vi "客户端侦听列表.vi"() -> ()   [LabVIEW 2016, in "wxpusher.lvlib"]
uses:
  wxpusher.lvlib
  <vilib>/Utility/miscctls.llb/LVPointTypeDef.ctl
  <vilib>/httpClient/LabVIEWHTTPClient.lvlib
panel:
  out "有效回调":refnum<k5>[](array[refnum])
  out "有效主机列表":T1(array[cluster])
  out "长度":i32
  out "错误输出":errorcluster
  out "数据输出":string
  in  "开机启动":bool
  out "remote port":u16
  out "remote address":string
  out "data out":string
  out "新增回调":refnum<k5>[](array[refnum])
  out "回调信息":T2
  out "新增主机列表":T1(array[cluster])
  in  "客户端列表":i32(listbox)
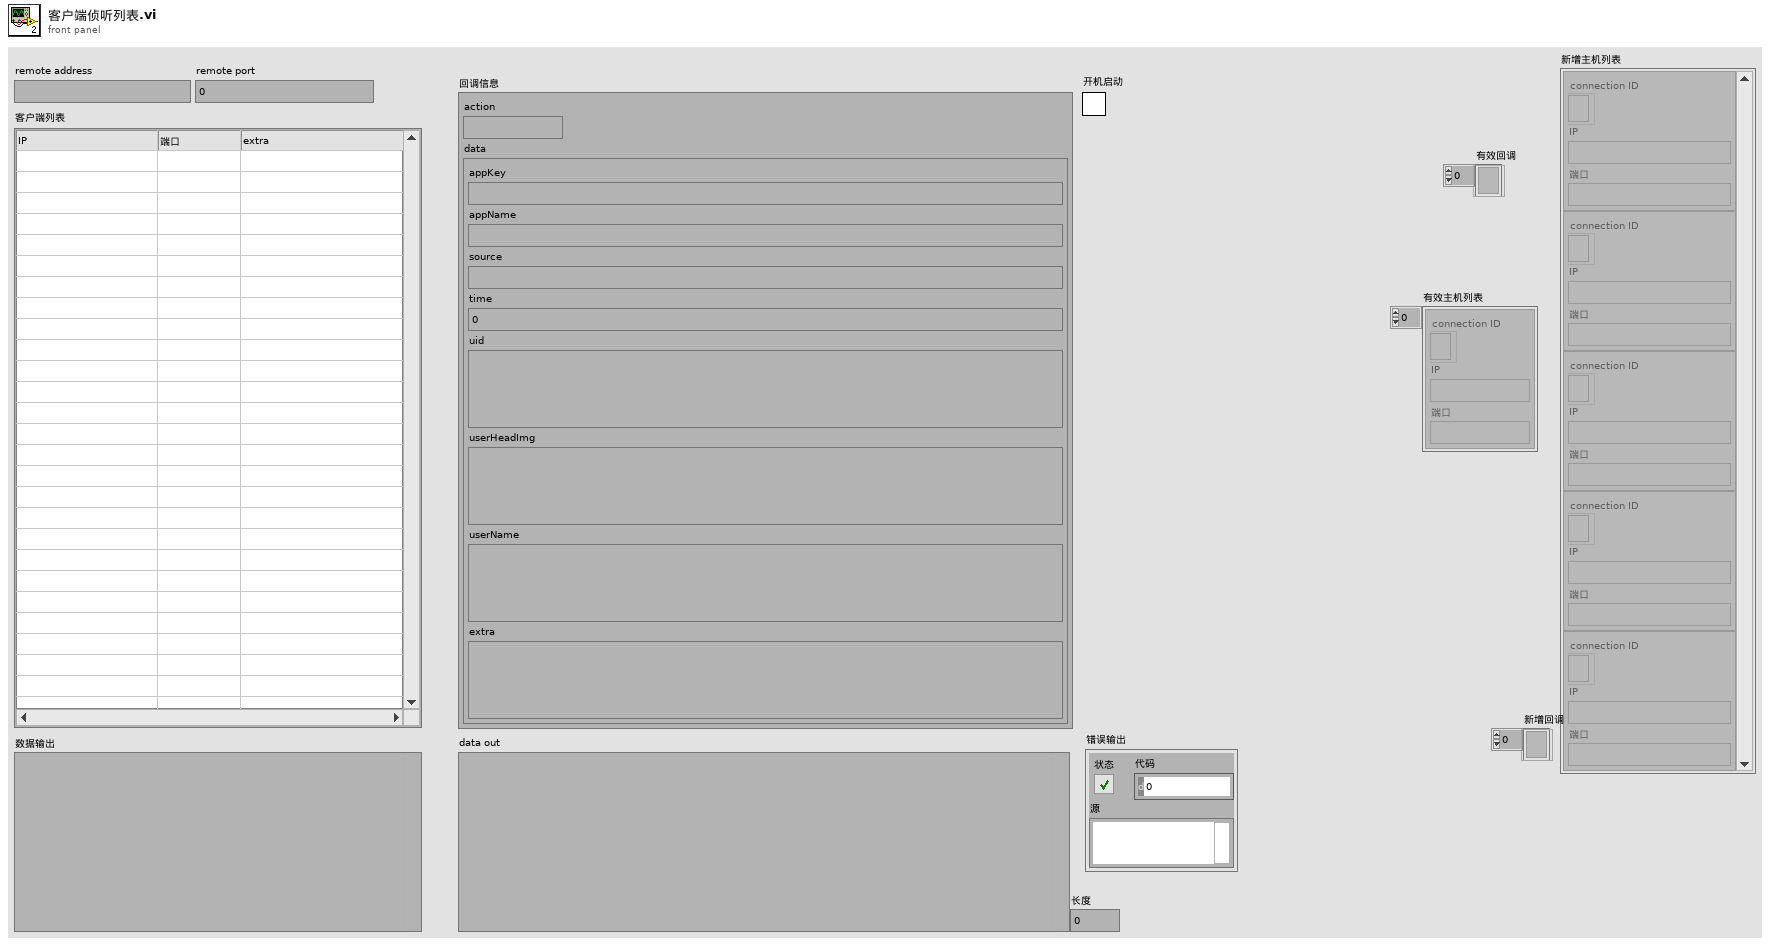
[diagram p1: front panel]
types:
  T1 = cluster{"connection ID":refnum<k5>, "IP":string, "端口":string}[]
  T2 = cluster{"action":string, "data":cluster{"appKey":string, "appName":string, "source":string, "time":u64, "uid":string, "userHeadImg":string, "userName":string, "extra":string}}
  T3 = typedef "LVPointTypeDef.ctl" = cluster{"Horizontal":i16, "Vertical":i16}
  T4 = cluster{"数据输出":string, "data":cluster{"action":string, "data":cluster{"appKey":string, "appName":string, "source":string, "time":u64, "uid":string, "userHeadImg":string, "userName":string, "extra":string}}}
  T5 = cluster{"connection ID":refnum<k5>, "IP":string, "端口":string}
  T6 = enum16{"Standard", "Buffered", "CRLF", "Immediate"}
  T7 = cluster{"cmd":string, "data":cluster{"png":u8[]}}
  T8 = typedef "LabVIEWHTTPClient.lvlib/ClientHandle.ctl" = refnum<k1>
  T9 = cluster{"data out":string, "类型和默认值":cluster{"action":string, "data":cluster{"appKey":string, "appName":string, "source":string, "time":u64, "uid":string, "userHeadImg":string, "userName":string, "extra":string}}}
  T10 = cluster{"cmd":string, "data":cluster{"action":string, "data":cluster{"appKey":string, "appName":string, "source":string, "time":u64, "uid":string, "userHeadImg":string, "userName":string, "extra":string}}}
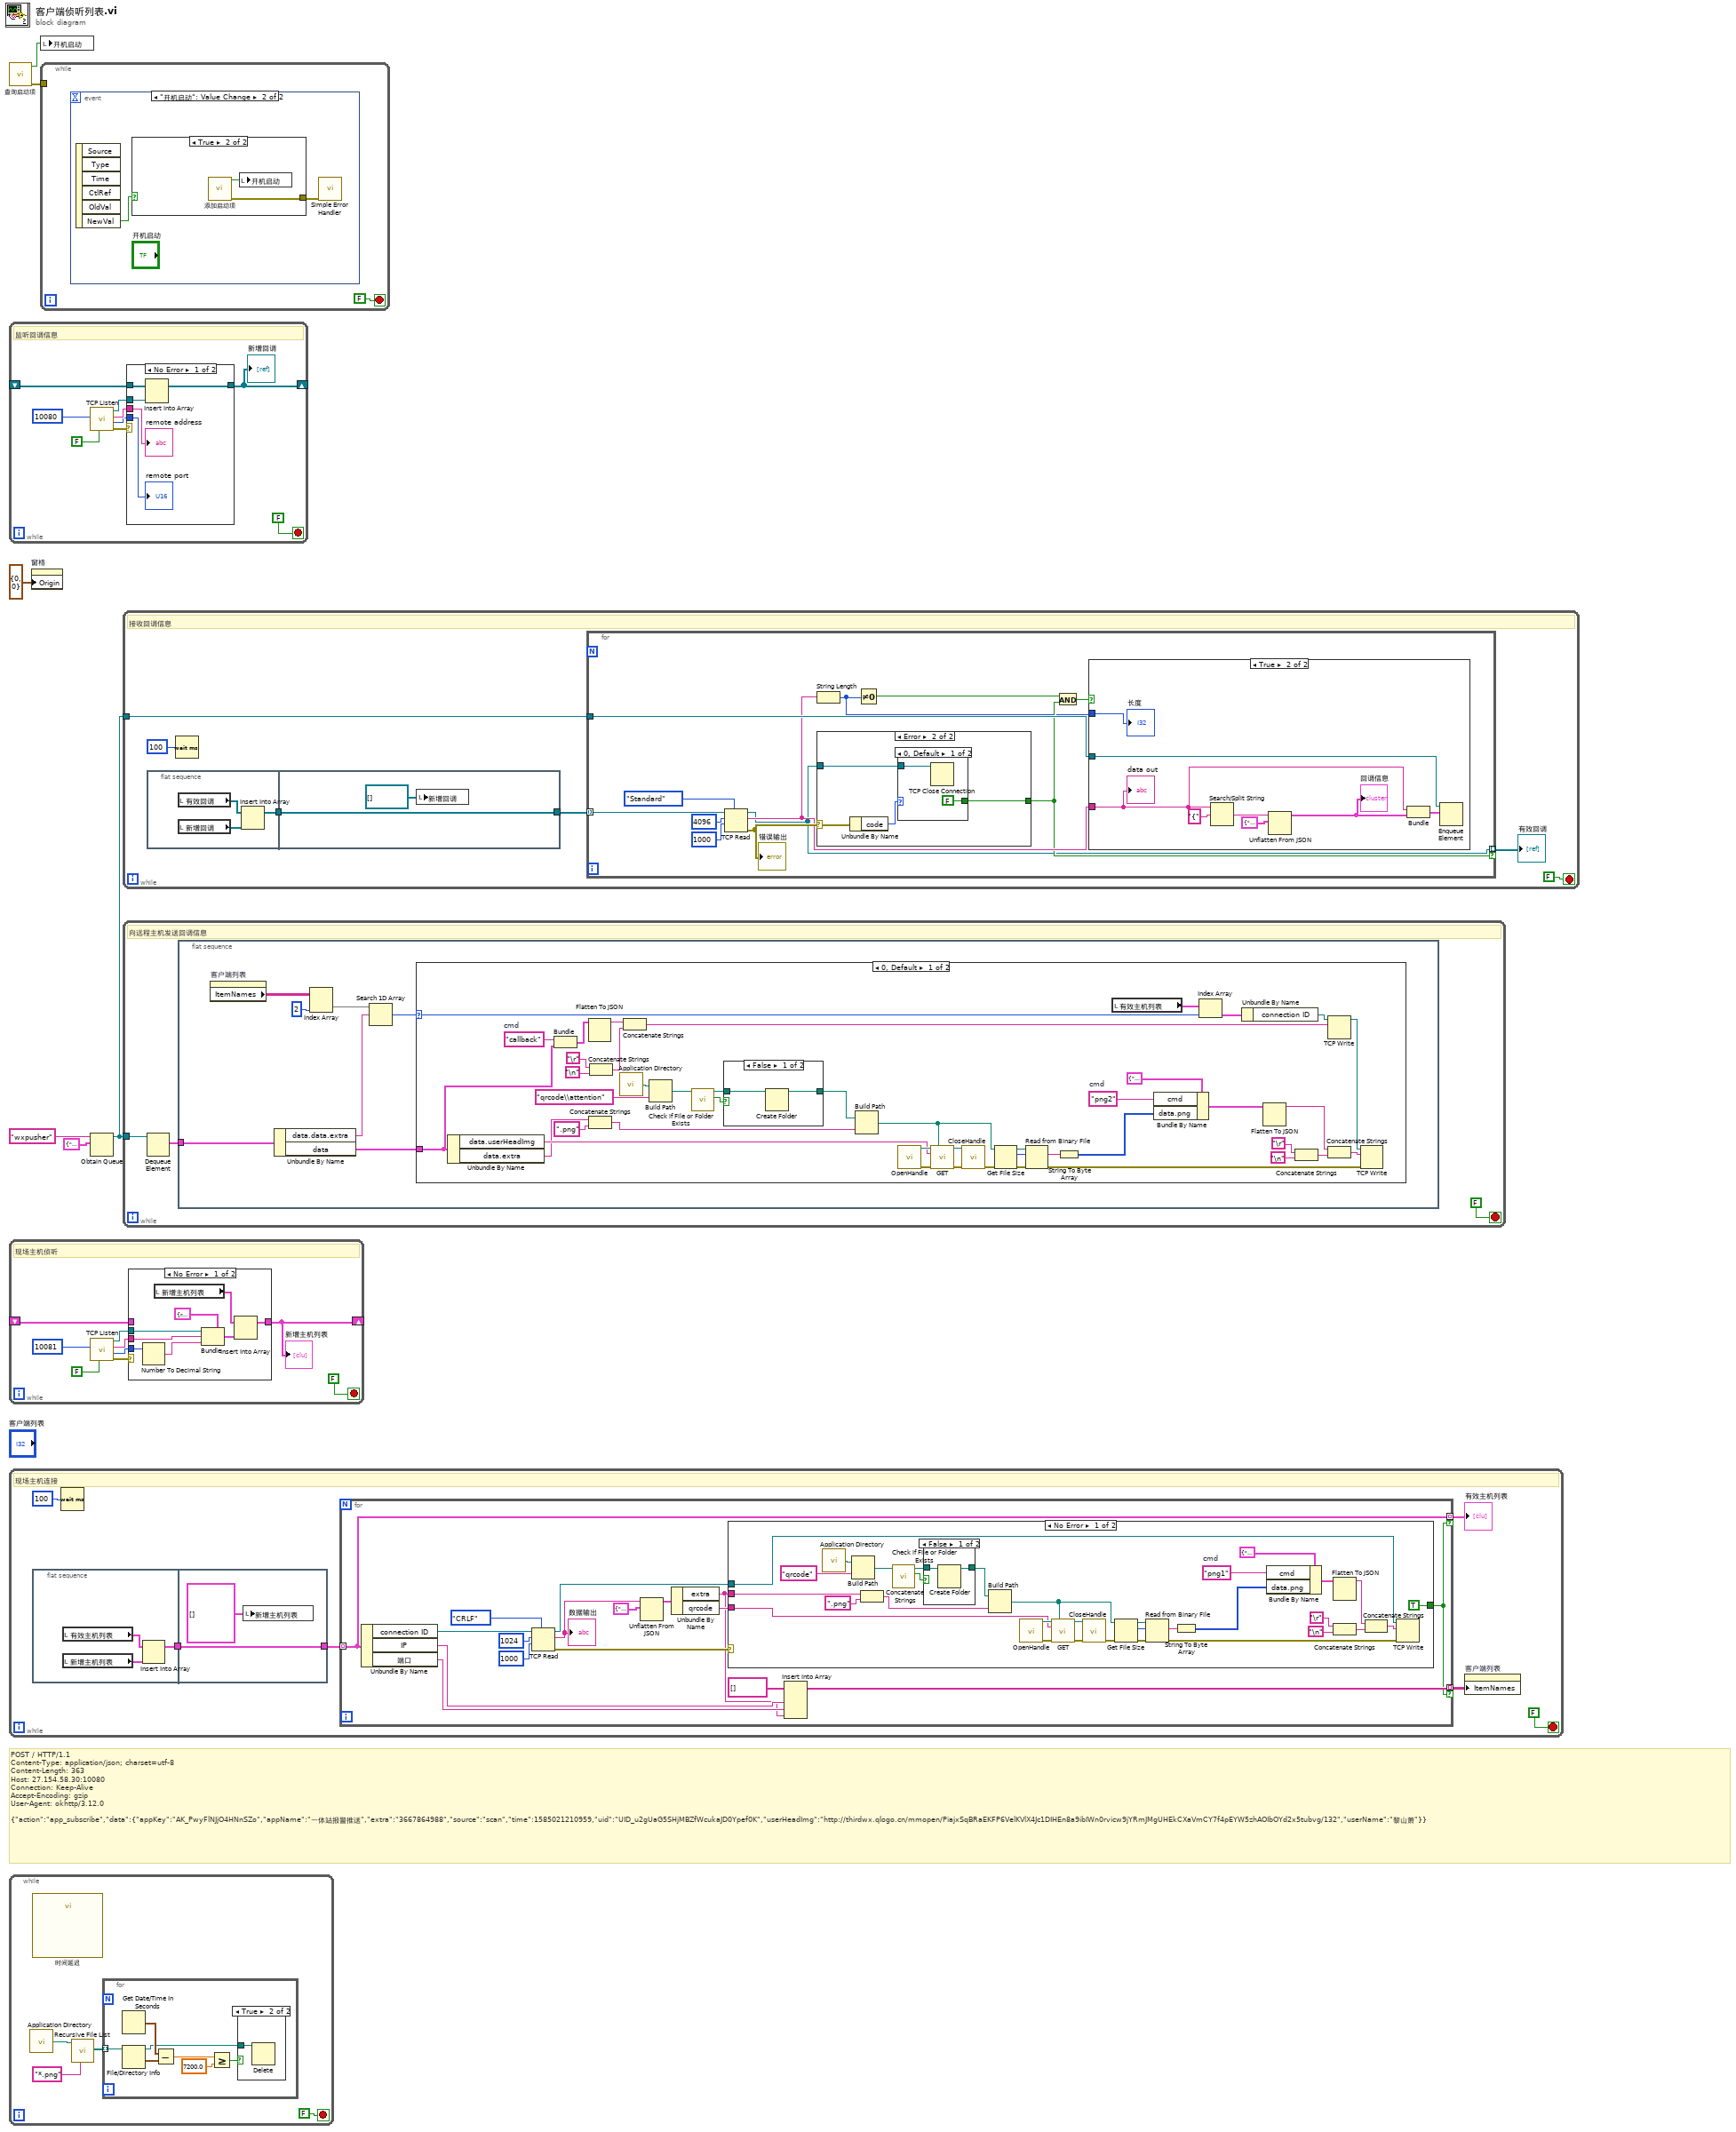
[diagram p0: block diagram]
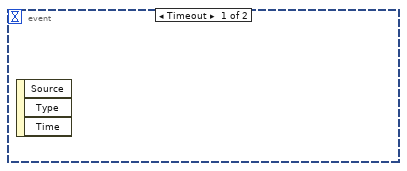
[diagram p3: hidden frame]
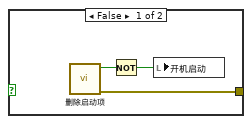
[diagram p4: hidden frame]
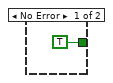
[diagram p6: hidden frame]
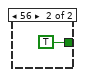
[diagram p7: hidden frame]
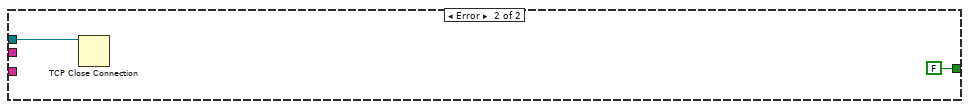
[diagram p12: hidden frame]
diagram:
  # "POST / HTTP/1.1\nContent-Type: application/json; charset=utf-8\nContent-Length: 363\nHost: 27.154.58.30:10080\nConnection: Keep-Alive\nAccept-Encoding: gzip\nUser-Agent: okhttp/3.12.0\n\n{\"action\":\"app_subscribe\",\"data\":{\"appKey\":\"AK_PwyFlNJjO4HNnSZo\",\"appName\":\"一体站报警推送\",\"extra\":\"3667864988\",\"source\":\"scan\",\"time\":1585021210959,\"uid\":\"UID_u2gUaG5SHjMBZfWcukaJD0Ypef0K\",\"userHeadImg\":\"http://thirdwx.qlogo.cn/mmopen/PiajxSqBRaEKFP6VelKVlX4Jc1DIHEn8a9ibIWn0rvicw9jYRmJMgUHEkCXaVmCY7f4pEYW5zhAOIbOYd2x5tubvg/132\",\"userName\":\"黎山萧\"}}"
  n1 = call "查询启动项.vi"() -> ("error out"=w3:errorcluster, "包含启动项"=w2:bool)  [unwired: 9 in, 1 out]
  n2 = while {
    shift-right: [w10] -> _
    shift-left: _ -> [w9]
    stop <- FALSE stop-if-true
    # "监听回调信息"
    n3 = call <vilib>:"TCP Listen.vi"("resolve remote address (T)"=FALSE, "port"=u16 10080) -> ("error out"=w13:errorcluster, "remote port"=w7:u16, "remote address"=w12:string, "connection ID"=w11:refnum<k5>)  [unwired: 5 in, 1 out]
    n4 = case shown="No Error" w13 {
      tunnel: w11 -> [w20 _]
      tunnel: w12 -> [w17 _]
      tunnel: [w19 w21] -> w10
      tunnel: w9 -> [w18 w21]
      tunnel: w7 -> [w16 _]
      frame No Error {
        n5 = Insert Into Array(array=w18, new element=w20) -> (w19:refnum<k5>[])  [unwired: 1 in]
        "remote address" <- w17
        "remote port" <- w16
      }
      frame Error {
      }
    }
    "新增回调" <- w10
  }
  n6 = while {
    shift-right: [w24] -> _
    shift-left: _ -> [w23]
    stop <- FALSE stop-if-true
    # "现场主机侦听"
    n7 = call <vilib>:"TCP Listen.vi"("resolve remote address (T)"=FALSE, "port"=u16 10081) -> ("error out"=w28:errorcluster, "remote port"=w25:u16, "remote address"=w26:string, "connection ID"=w27:refnum<k5>)  [unwired: 5 in, 1 out]
    n8 = case shown="No Error" w28 {
      tunnel: w27 -> [w38 _]
      tunnel: w26 -> [w32 _]
      tunnel: w25 -> [w33 _]
      tunnel: [w36 w39] -> w24
      tunnel: w23 -> [_ w39]
      frame No Error {
        n9 = Number To Decimal String(number=w33) -> (decimal integer string=w35:string)  [unwired: 1 in]
        n10 = local read "新增主机列表"() -> (w31:T1)
        n11 = Bundle(cluster=T5 {"connection ID"=refnum, "IP"="", "端口"=""} ("簇"), "connection ID"=w38, "IP"=w32, "端口"=w35) -> (w37:T5)
        n12 = Insert Into Array(array=w31, new element=w37) -> (w36:T1)  [unwired: 1 in]
      }
      frame Error {
      }
    }
    "新增主机列表" <- w24
  }
  n13 = while {
    stop <- FALSE stop-if-true
    # "现场主机连接"
    n14 = flat-sequence {
      tunnel: [w46] -> w40
      tunnel: [w50] -> w42
      tunnel: w40 -> [w50]
      frame #0 {
        n15 = local read "有效主机列表"() -> (w47:T1)
        n16 = local read "新增主机列表"() -> (w48:T1)
        n17 = Insert Into Array(array=w47, new element=w48) -> (w46:T1)  [unwired: 1 in]
      }
      frame #1 {
        n18 = local write "新增主机列表"(T1 [] ("新增主机列表")) -> ()
      }
    }
    n19 = Wait (ms)(milliseconds to wait=u32 100 ("等待时间（毫秒）")) -> ()  [unwired: 1 out]
    n20 = for {
      tunnel: w42 -> [w56] mode=indexing
      tunnel: [w61] -> w43 mode=indexing if=w55
      tunnel: [w56] -> w41 mode=indexing if=w55
      n21 = Unbundle By Name(w56) -> ("connection ID"=w67:refnum<k5>, "IP"=w64:string, "端口"=w63:string)
      n22 = TCP Read(connection ID=w67, bytes to read=1024 ("读取的字节"), 7:T6."CRLF" ("模式（标准）"), 9:1000 ("超时毫秒(25000)")) -> (connection ID out=w54:refnum<k5>, data out=w59:string, error out=w60:errorcluster)  [unwired: 1 in]
      "数据输出" <- w59
      n23 = Unflatten From JSON(JSON string=w59, type and defaults=cluster{"extra":string, "qrcode":string} {"extra"="", "qrcode"=""}) -> (value=w57:cluster{"extra":string, "qrcode":string})  [unwired: 5 in, 1 out]
      n24 = Unbundle By Name(w57) -> ("extra"=w52:string, "qrcode"=w53:string)
      n25 = case shown="No Error" w60 {
        tunnel: [TRUE FALSE] -> w55
        tunnel: w54 -> [w70 w103]
        tunnel: w53 -> [w69 _]
        tunnel: w52 -> [w68 _]
        frame No Error {
          w96 = "png1"  # cmd
          n26 = call <vilib>:"Application Directory.vi"() -> ("Application Directory"=w88:path)
          n27 = Build Path(base path=w88, name or relative path="qrcode" ("名称或相对路径")) -> (appended path=w76:path)
          n28 = Concatenate Strings(w68, ".png" ("字符串")) -> (w81:string)
          n29 = call <vilib>:"Check if File or Folder Exists.vi"("path"=w76) -> ("file or folder exists?"=w78:bool, "dup path"=w77:path)  [unwired: 8 in, 1 out]
          n30 = case shown="False" w78 {
            tunnel: [w101 w102] -> w75
            tunnel: w77 -> [w100 w102]
            frame False {
              n31 = Create Folder(path (use dialog)=w100) -> (created path=w101:path)  [unwired: 2 in, 2 out]
            }
            frame True {
            }
          }
          n32 = Build Path(base path=w75, name or relative path=w81) -> (appended path=w82:path)
          n33 = call <vilib>:"OpenHandle.vi"() -> ("client handle out"=w71:T8, "error out"=w72:errorcluster)  [unwired: 14 in]
          n34 = call <vilib>:"GET.vi"("client handle"=w71, "output file"=w82, "url"=w69, "error in (no error)"=w72) -> ("client handle out"=w73:T8, "error out"=w74:errorcluster)  [unwired: 8 in, 2 out]
          n35 = call <vilib>:"CloseHandle.vi"("client handle"=w73, "error in (no error)"=w74) -> ("error out"=w84:errorcluster)  [unwired: 13 in]
          n36 = Get File Size(file=w82, error in=w84) -> (refnum out=w83:refnum<file>, size (in bytes)=w86:i64, 0:w85:errorcluster)
          n37 = Read from Binary File(8:w85, 10:w86, 11:w83) -> (0:w87:errorcluster, 2:w97:string)  [unwired: 3 in, 2 out]
          n38 = String To Byte Array(string=w97) -> (unsigned byte array=w98:u8[])
          n39 = Bundle By Name(cluster=T7 {"cmd"="", "data"={"png"=[]}}, "cmd"=w96, "data.png"=w98) -> (w90:T7)
          n40 = Flatten To JSON(anything=w90) -> (JSON string=w91:string)  [unwired: 2 in, 1 out]
          n41 = Concatenate Strings("\r", "\n") -> (w95:string)
          n42 = Concatenate Strings(w91, w95) -> (w92:string)
          n43 = TCP Write(connection ID=w70, data in=w92, error in (no error)=w87) -> ()  [unwired: 1 in, 3 out]
        }
        frame Error {
          n44 = TCP Close Connection(connection ID=w103) -> ()  [unwired: 2 in, 2 out]
        }
      }
      n45 = Insert Into Array(array=string[] [] ("数组"), new element #1=w64, new element #2=w63, new element #3=w52) -> (w61:string[])  [unwired: 1 in]
    }
    "有效主机列表" <- w41
    n46 = property on="客户端列表" class="MCListbox (strict)"("ItemNames"=w43) -> ()  [unwired: 2 in, 2 out]
  }
  n47 = while {
    stop <- FALSE stop-if-true
    n48 = call <vilib>:"Application Directory.vi"() -> ("Application Directory"=w107:path)
    n49 = call "时间延迟"() -> ()  [unwired: 11 in, 1 out]
    n50 = call <vilib>:"Recursive File List.vi"("pattern"="*.png", "Folder Path"=w107) -> ("All Files in Dir"=w105:path[])  [unwired: 5 in, 4 out]
    n51 = for {
      tunnel: w105 -> [w115] mode=indexing
      n52 = Get Date/Time In Seconds() -> (seconds since 1Jan1904=w113:timestamp)
      n53 = File/Directory Info(path=w115) -> (path out=w109:path, last mod=w114:timestamp)  [unwired: 1 in, 5 out]
      n54 = Subtract(x=w113, y=w114) -> (x-y=w112:dbl)
      n55 = Greater Or Equal?(x=w112, y=7200.0) -> (x >= y?=w110:bool)
      n56 = case shown="True" w110 {
        tunnel: w109 -> [_ w116]
        frame False {
        }
        frame True {
          n57 = Delete(path (use dialog)=w116) -> ()  [unwired: 4 in, 3 out]
        }
      }
    }
  }
  n58 = property on="窗格" class="Pane"("Origin"=T3 {"Horizontal"=0, "Vertical"=0} ("原点")) -> ()  [unwired: 2 in, 2 out]
  n59 = local write "开机启动"(w2) -> ()
  n60 = while {
    tunnel: w3 -> [_]
    stop <- FALSE stop-if-true
    n61 = event shown="[1] \"开机启动\": Value Change" {
      selector: _ -> [_ _]
      dyn-events: _ -> [_ _]
      timeout: _ -> [_ _]
      event Timeout {
        n62 = event-data() -> ()  [unwired: 1 in, 3 out]
      }
      event "开机启动": Value Change {
        n63 = event-data() -> ("NewVal"=w119:bool)  [unwired: 1 in, 5 out]
        n64 = case shown="True" w119 {
          tunnel: [w120 w123] -> w118
          frame False {
            n65 = call "删除启动项.vi"() -> ("error out"=w120:errorcluster, "删除标记"=w122:bool)  [unwired: 10 in]
            n66 = Not(x=w122) -> (.not. x?=w121:bool)
            n67 = local write "开机启动"(w121) -> ()
          }
          frame True {
            n68 = call "添加启动项.vi"() -> ("error out"=w123:errorcluster, "添加成功标记"=w124:bool)  [unwired: 10 in]
            n69 = local write "开机启动"(w124) -> ()
          }
        }
        n70 = call <vilib>:"Simple Error Handler.vi"("error in (no error)"=w118) -> ()  [unwired: 4 in, 5 out]
      }
    }
  }
  n71 = Obtain Queue(name (unnamed)="wxpusher" ("名称（未命名）"), element data type=T4 {"数据输出"="", "data"={"action"="", "data"={"appKey"="", "appName"="", "source"="", "time"=0, "uid"="", "userHeadImg"="", "userName"="", "extra"=""}}}) -> (queue out=w4:refnum<queue>)  [unwired: 3 in, 2 out]
  n72 = while "While循环" {
    tunnel: w4 -> [w129]
    stop <- FALSE stop-if-true
    # "接收回调信息"
    n73 = flat-sequence {
      tunnel: [w131] -> w125
      tunnel: [w135] -> w126
      tunnel: w125 -> [w135]
      frame #0 {
        n74 = local read "有效回调"() -> (w133:refnum<k5>[])
        n75 = local read "新增回调"() -> (w132:refnum<k5>[])
        n76 = Insert Into Array(array=w133, new element=w132) -> (w131:refnum<k5>[])  [unwired: 1 in]
      }
      frame #1 {
        n77 = local write "新增回调"(refnum<k5>[] [] ("新增回调")) -> ()
      }
    }
    n78 = Wait (ms)(milliseconds to wait=u32 100 ("等待时间（毫秒）")) -> ()  [unwired: 1 out]
    n79 = for {
      tunnel: w129 -> [w147]
      tunnel: w126 -> [w143] mode=indexing
      tunnel: [w137] -> w127 mode=indexing if=w138
      n80 = TCP Read(connection ID=w143, bytes to read=4096 ("读取的字节"), 7:T6."Standard" ("模式（标准）"), 9:1000 ("超时毫秒(25000)")) -> (connection ID out=w137:refnum<k5>, data out=w141:string, error out=w142:errorcluster)  [unwired: 1 in]
      "错误输出" <- w142
      n81 = String Length(string=w141) -> (length=w136:i32)
      n82 = case shown="Error" w142 {
        selector: w142 -> [_ w160]
        tunnel: [TRUE w158] -> w138
        tunnel: w137 -> [_ w157]
        frame No Error {
        }
        frame Error {
          n83 = Unbundle By Name(w160) -> ("code"=w159:i32)
          n84 = case shown="0, Default" w159 {
            tunnel: [FALSE TRUE] -> w158
            tunnel: w157 -> [w161 _]
            frame 0, Default {
              n85 = TCP Close Connection(connection ID=w161) -> ()  [unwired: 2 in, 2 out]
            }
            frame 56 {
            }
          }
        }
      }
      n86 = Not Equal To 0?(x=w136) -> (x != 0?=w139:bool)
      n87 = And(x=w139, y=w138) -> (x .and. y?=w140:bool)
      n88 = case shown="True" w140 {
        tunnel: w147 -> [_ w155]
        tunnel: w141 -> [_ w154]
        tunnel: w136 -> [_ w148]
        frame False {
        }
        frame True {
          n89 = Search/Split String(string=w154, search string/char (-)="{" ("搜索字符串/字符(-)")) -> (match + rest of string=w151:string)  [unwired: 1 in, 2 out]
          n90 = Unflatten From JSON(JSON string=w151, type and defaults=T2 {"action"="", "data"={"appKey"="", "appName"="", "source"="", "time"=0, "uid"="", "userHeadImg"="", "userName"="", "extra"=""}} ("类型和默认值")) -> (value=w150:T2)  [unwired: 5 in, 1 out]
          "回调信息" <- w150
          n91 = Bundle("data out"=w154, "类型和默认值"=w150) -> (w149:T9)  [unwired: 1 in]
          n92 = Enqueue Element(queue=w155, element=w149) -> ()  [unwired: 2 in, 3 out]
          "data out" <- w154
          "长度" <- w148
        }
      }
    }
    "有效回调" <- w127
  }
  n93 = while {
    tunnel: w4 -> [w166]
    stop <- FALSE stop-if-true
    # "向远程主机发送回调信息"
    n94 = Dequeue Element(queue=w166) -> (element=w164:T4)  [unwired: 2 in, 3 out]
    n95 = flat-sequence {
      tunnel: w164 -> [w173]
      frame #0 {
        n96 = property on="客户端列表" class="MCListbox (strict)"() -> ("ItemNames"=w172:string[][])  [unwired: 2 in, 2 out]
        n97 = Unbundle By Name(w173) -> ("data.data.extra"=w169:string, "data"=w167:T2)
        n98 = Index Array(array=w172, index (col)=2 ("禁用的索引 (列)")) -> (element=w170:string[])  [unwired: 1 in]
        n99 = Search 1D Array(1D array=w170, element=w169) -> (index of element=w168:i32)  [unwired: 1 in]
        n100 = case shown="0, Default" w168 {
          selector: w168 -> [w215 _]
          tunnel: w167 -> [w207 _]
          frame 0, Default {
            w179 = "png2"  # cmd
            w206 = "callback"  # cmd
            n101 = Unbundle By Name(w207) -> ("data.userHeadImg"=w176:string, "data.extra"=w175:string)
            n102 = Bundle("cmd"=w206, "data"=w207) -> (w205:T10)  [unwired: 1 in]
            n103 = Flatten To JSON(anything=w205) -> (JSON string=w212:string)  [unwired: 2 in, 1 out]
            n104 = Concatenate Strings(w175, ".png" ("字符串")) -> (w194:string)
            n105 = Concatenate Strings("\r", "\n") -> (w208:string)
            n106 = call <vilib>:"Application Directory.vi"() -> ("Application Directory"=w187:path)
            n107 = Concatenate Strings(w212, w208) -> (w211:string)
            n108 = Build Path(base path=w187, name or relative path="qrcode\\attention" ("名称或相对路径")) -> (appended path=w199:path)
            n109 = call <vilib>:"Check if File or Folder Exists.vi"("path"=w199) -> ("file or folder exists?"=w197:bool, "dup path"=w198:path)  [unwired: 8 in, 1 out]
            n110 = case shown="False" w197 {
              tunnel: [w218 w219] -> w200
              tunnel: w198 -> [w217 w219]
              frame False {
                n111 = Create Folder(path (use dialog)=w217) -> (created path=w218:path)  [unwired: 2 in, 2 out]
              }
              frame True {
              }
            }
            n112 = Build Path(base path=w200, name or relative path=w194) -> (appended path=w193:path)
            n113 = call <vilib>:"OpenHandle.vi"() -> ("client handle out"=w204:T8, "error out"=w203:errorcluster)  [unwired: 14 in]
            n114 = call <vilib>:"GET.vi"("client handle"=w204, "output file"=w193, "url"=w176, "error in (no error)"=w203) -> ("client handle out"=w202:T8, "error out"=w201:errorcluster)  [unwired: 8 in, 2 out]
            n115 = call <vilib>:"CloseHandle.vi"("client handle"=w202, "error in (no error)"=w201) -> ("error out"=w191:errorcluster)  [unwired: 13 in]
            n116 = Get File Size(file=w193, error in=w191) -> (refnum out=w192:refnum<file>, size (in bytes)=w189:i64, 0:w190:errorcluster)
            n117 = Read from Binary File(8:w190, 10:w189, 11:w192) -> (0:w188:errorcluster, 2:w178:string)  [unwired: 3 in, 2 out]
            n118 = String To Byte Array(string=w178) -> (unsigned byte array=w177:u8[])
            n119 = local read "有效主机列表"() -> (w216:T1)
            n120 = Bundle By Name(cluster=T7 {"cmd"="", "data"={"png"=[]}}, "cmd"=w179, "data.png"=w177) -> (w185:T7)
            n121 = Index Array(array=w216, index=w215) -> (element=w214:T5)
            n122 = Unbundle By Name(w214) -> ("connection ID"=w213:refnum<k5>)
            n123 = Flatten To JSON(anything=w185) -> (JSON string=w184:string)  [unwired: 2 in, 1 out]
            n124 = Concatenate Strings("\r", "\n") -> (w180:string)
            n125 = TCP Write(connection ID=w213, data in=w211) -> (connection ID out=w174:refnum<k5>)  [unwired: 2 in, 2 out]
            n126 = Concatenate Strings(w184, w180) -> (w183:string)
            n127 = TCP Write(connection ID=w174, data in=w183, error in (no error)=w188) -> ()  [unwired: 1 in, 3 out]
          }
          frame -1 {
          }
        }
      }
    }
  }
